vi "UnifiedCameraCalibration.vi"(5 "um/pix conversion method":T5 items=["Strip Centers", "Signal Fit, Left to Right", "Projection + Signal Fit"], 7 "Sharpness assessment method":T4, 8 "error in (no error)":errorcluster, 10 "Naming Convention":string="*.png", 11 "Images Directory":path=path "C:/Users/sciollalab/cernbox/BNL/Datasets/AutofocusStrips") -> (0 "error out":errorcluster, 3 "Camera calibration results":T2 {"Working distance to stave [mm]" format="%#_13g"})   [LabVIEW 2016]
uses:
  Utils/Enum_TypeDefinitions/Enum_TypeDef_ImageSharpnessAnalysisMethod.ctl
  Utils/Enum_TypeDefinitions/Enum_TypeDef_CameraCalibrationResults.ctl
  Utils/Enum_TypeDefinitions/Ring_TypeDef_PixUmConversionMethod.ctl
  <vilib>/Utility/file.llb/Read Delimited Spreadsheet (DBL).vi
panel:
  out "Processing Image #":i32
  in  "Tab Control":T1(tab)
  out "Sharpness vs Height":T3(graph)
  out "Uncertainty on height":dbl
  out "Optimized height":dbl
  out "Conversion vs Height":cluster{"all rows":dbl[], dbl[]}[](graph)
  out "Conversion [um/pix]":dbl
  out "Uncertainty on conversion":dbl
  # "CALIBRATE CAMERA Brandeis University - Brookhaven National Laboratory * ATLAS Phase II Inner Tracker Upgrade"
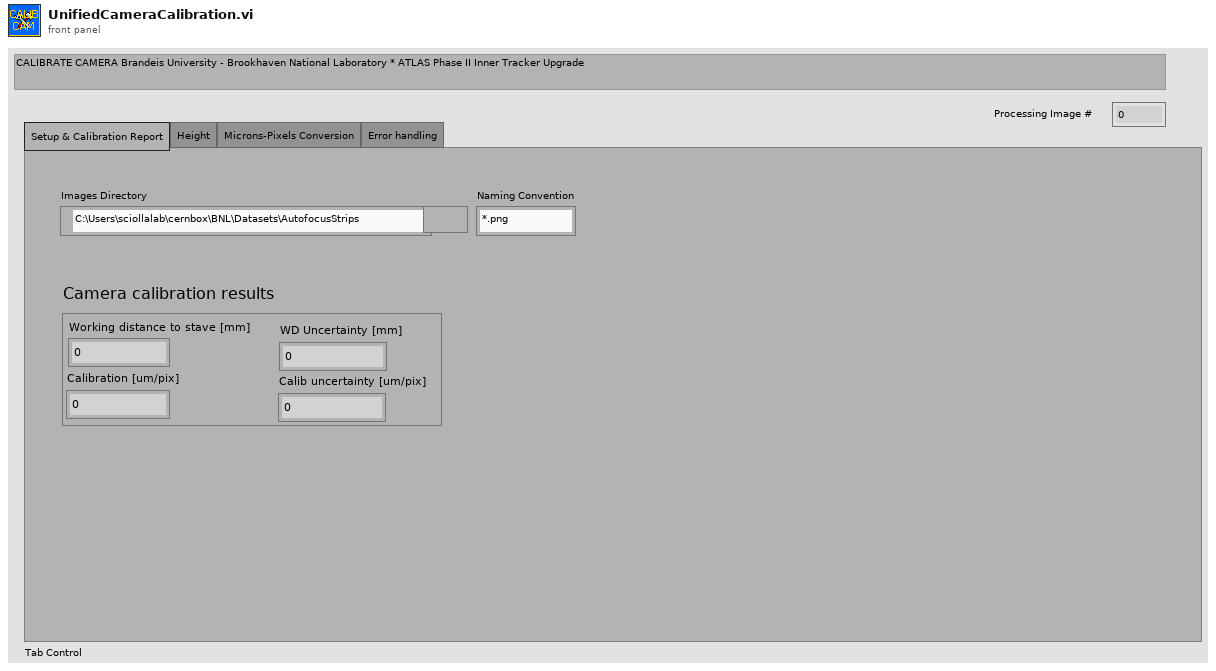
[diagram p1: front panel]
types:
  T1 = enum32{"Setup & Calibration Report", "Height", "Microns-Pixels Conversion", "Error handling"}
  T2 = typedef "Enum_TypeDef_CameraCalibrationResults.ctl" = cluster{"Working distance to stave [mm]":dbl, "WD Uncertainty [mm]":dbl, "Calibration [um/pix]":dbl, "Calib uncertainty [um/pix]":dbl}
  T3 = cluster{"Radius bins":dbl[], "Best Gaussian Fit":dbl[]}[]
  T4 = typedef "Enum_TypeDef_ImageSharpnessAnalysisMethod.ctl" = enum16{"RMS( Intensity )", "Mean( Laplacian Convolution )"}
  T5 = typedef "Ring_TypeDef_PixUmConversionMethod.ctl" = u16
  T6 = typedef "Image Type" = u32
  T7 = typedef "IMAQ Image.ctl" = refnum<image>
  T8 = typedef "Graph_TypeDef_XY.ctl" = cluster{"Radius bins":dbl[], "Best Gaussian Fit":dbl[]}[]
  T9 = cluster{"Optimized position":dbl, "Uncertainty on position":dbl, "Mean y":dbl, "Mean of y uncertainties":dbl}
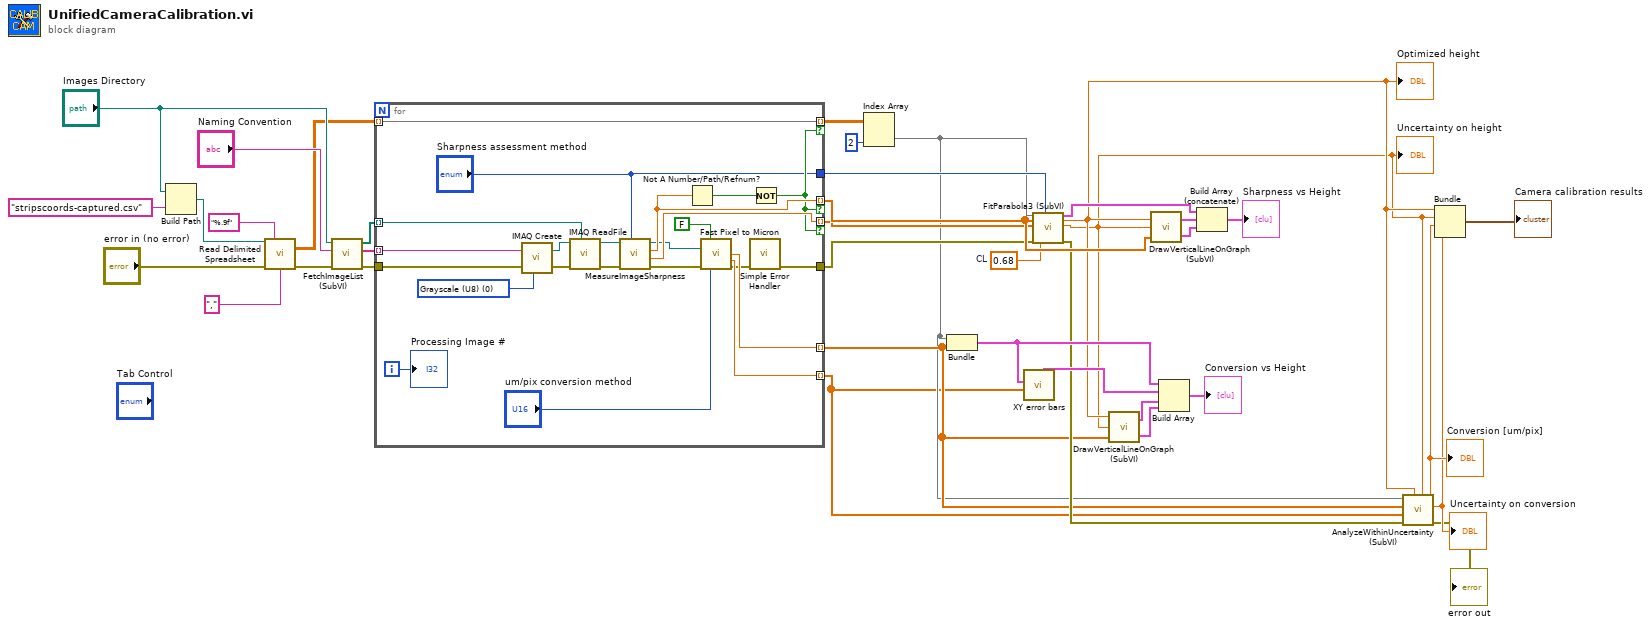
[diagram p0: block diagram]
diagram:
  w16 = 0.68  # CL
  n1 = Build Path(base path="Images Directory", name or relative path="stripscoords-captured.csv") -> (appended path=w36:path)
  n2 = call-poly <vilib>:"Read Delimited Spreadsheet.vi"("file path (dialog if empty)"=w36, "format (%.3f)"="%.9f", "error in (no error)"="error in (no error)", "delimiter (\\t)"="," ("delimiter (\\t)")) -> ("all rows"=w26:dbl[][], "error out"=w30:errorcluster)  [unwired: 6 in, 4 out]
  n3 = call "FetchImageList (SubVI).vi"("error in (no error)"=w30, "Naming Convention"="Naming Convention", "Images Directory"="Images Directory") -> ("error out"=w37:errorcluster, "List of Image Names"=w27:string[], "List of Image Paths"=w38:path[])  [unwired: 5 in, 1 out]
  n4 = for {
    tunnel: w38 -> [w58] mode=indexing
    tunnel: w27 -> [w61] mode=indexing
    tunnel: w37 -> [w57]
    tunnel: [w48] -> w17 mode=indexing if=w46
    tunnel: [w53] -> w15 mode=indexing if=w46
    tunnel: [w52] -> w5 mode=indexing
    tunnel: [w51] -> w3 mode=indexing
    tunnel: w26 -> [w49] mode=indexing
    tunnel: [w49] -> w25 mode=indexing if=w46
    tunnel: [w42] -> w14
    tunnel: ["Sharpness assessment method"] -> w13
    i -> [w50]
    w54 = T6 0 items=["Grayscale (U8)", "Grayscale (I16)", "Grayscale (SGL)", "Complex (CSG)", "RGB (U32)", "HSL (U32)", "RGB (U64)", "Grayscale (U16)"] ("Image Type")
    n5 = call "IMAQ Create"("Image Name"=w61, "Image Type"=w54, "error in (no error)"=w57) -> ("New Image"=w59:T7, "error out"=w60:errorcluster)  [unwired: 2 in]
    n6 = call "IMAQ ReadFile"("File Path"=w58, "error in (no error)"=w60, "Image"=w59) -> ("error out"=w56:errorcluster, "Image Out"=w41:T7)  [unwired: 4 in, 3 out]
    n7 = call "MeasureImageSharpness.vi"("Method"="Sharpness assessment method", "error in (no error)"=w56, "Image In"=w41) -> ("error out"=w55:errorcluster, "Sharpness Uncertainty"=w53:dbl, "Sharpness"=w48:dbl, "Image Out"=w40:T7)  [unwired: 5 in]
    n8 = Not A Number/Path/Refnum?(number/path/refnum=w48) -> (NaN/Path/Refnum?=w47:bool)
    n9 = call "Fast Pixel to Micron.vi"("Testing?"=FALSE, "External Image In"=w40, "error in (no error)"=w55, "Conversion Method"="um/pix conversion method") -> ("Corrected um/pix"=w52:dbl, "Corrected um/pix uncertainty"=w51:dbl, "error out"=w43:errorcluster)  [unwired: 5 in, 4 out]
    n10 = call <vilib>:"Simple Error Handler.vi"("error in (no error)"=w43) -> ("error out"=w42:errorcluster)  [unwired: 4 in, 4 out]
    n11 = Not(x=w47) -> (.not. x?=w46:bool)
    "Processing Image #" <- w50
  }
  n12 = Index Array(array=w25, index (col)=2 ("disabled index (col)")) -> (element=w4:dbl[])  [unwired: 1 in]
  n13 = Bundle("all rows"=w4, w5) -> (w12:cluster{"all rows":dbl[], dbl[]})  [unwired: 1 in]
  n14 = call "XY error bars.vi"("XY plot"=w12, "Xerror"=w3) -> ("Y error bars"=w11:cluster{dbl[], dbl[]})  [unwired: 6 in, 2 out]
  n15 = call "FitParabola3 (SubVI).vi"("x values"=w4, "y values"=w17, "delta y values"=w15, "error in"=w14, "confidence level"=w16, "Poly fit algorithm"=w13) -> ("Plot"=w24:T8, "Optimized position"=w10:dbl, "Uncertainty on position"=w9:dbl, "error out"=w6:errorcluster)  [unwired: 10 in]
  "Uncertainty on height" <- w9
  "Optimized height" <- w10
  n16 = call "DrawVerticalLineOnGraph (SubVI).vi"("Array"=w5, "value uncertainty"=w9, "x = value"=w10) -> ("X error bars"=w21:cluster{dbl[], dbl[]}, "Line at x = value"=w22:cluster{dbl[], dbl[]})
  n17 = call "DrawVerticalLineOnGraph (SubVI).vi"("Array"=w17, "value uncertainty"=w9, "x = value"=w10) -> ("X error bars"=w19:cluster{dbl[], dbl[]}, "Line at x = value"=w20:cluster{dbl[], dbl[]})
  n18 = Build Array(w12, w11, w22, w21) -> (→"Conversion vs Height":cluster{"all rows":dbl[], dbl[]}[])
  n19 = Build Array (concatenate)(w24, w20, w19) -> (→"Sharpness vs Height":T8)
  n20 = call "AnalyzeWithinUncertainty (SubVI).vi"("Uncertainty on mean x"=w9, "Mean x"=w10, "error in (no error)"=w6, "y uncertainties"=w3, "y values"=w5, "x values"=w4) -> ("error out"=→"error out":errorcluster, "Mean of y uncertainties"=w7:dbl, "Mean y"=w8:dbl)  [unwired: 3 in]
  "Conversion [um/pix]" <- w8
  "Uncertainty on conversion" <- w7
  n21 = Bundle("Optimized position"=w10, "Uncertainty on position"=w9, "Mean y"=w8, "Mean of y uncertainties"=w7) -> (→"Camera calibration results":T9)  [unwired: 1 in]
